vi "Read N channels.vi"(8 "error in (no error)":errorcluster, 11 "device data model in":refnum<class "ET-7016i Data Model.lvclass">) -> (0 "error out":errorcluster, 2 "N channel":T1, 3 "device data model out":refnum<class "ET-7016i Data Model.lvclass">)   [LabVIEW 2021, in "ET-7016i Data Model.lvclass"]
doc: "Retrieves objects from the device model."
uses:
  ET-7016i Data Model.lvclass
  ET-7016i Data Model.lvclass/ET-7016i Data Model.ctl
  N channel.ctl
  Device Data Model.lvclass
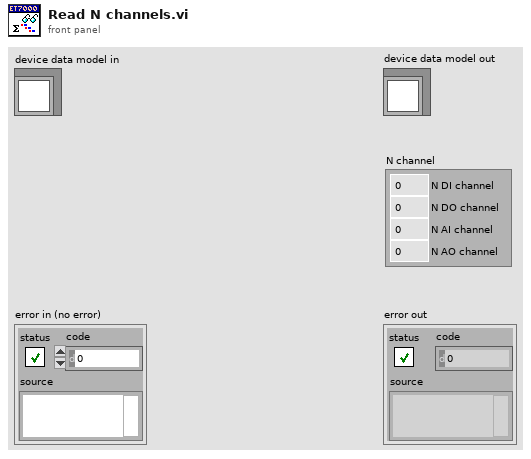
[diagram p1: front panel]
types:
  T1 = typedef "Device Data Model.lvclass/N channel.ctl" = cluster{"N DI channel":i32, "N DO channel":i32, "N AI channel":i32, "N AO channel":i32}
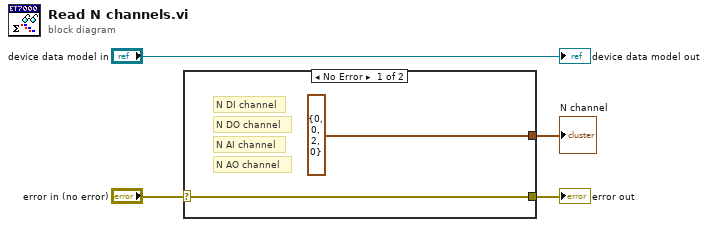
[diagram p0: block diagram]
diagram:
  n1 = case shown="No Error" "error in (no error)" {
    selector: "error in (no error)" -> [w5 w7]
    tunnel: [w5 w7] -> w3
    tunnel: [T1 {"N DI channel"=0, "N DO channel"=0, "N AI channel"=2, "N AO channel"=0} ("N channel") _] -> w1
    frame No Error {
      # "N AO channel"
      # "N AI channel"
      # "N DO channel"
      # "N DI channel"
    }
    frame Error {
    }
  }
  "error out" <- w3
  "N channel" <- w1
  "device data model out" <- "device data model in"
